vi "To XML - Invalid character in Message - XML does not contain invalid character.vi"() -> ()   [LabVIEW 2013, in "JUnit XML Tests.lvlib" / "Test Case.lvlib"]
uses:
  Test Case.lvlib
  JUnit XML/Test Case/Test Case.lvclass
  <vilib>/addons/_JKI Toolkits/Caraya/classes/Assert/Assert Equal Value_Variant.vi
  <vilib>/addons/_JKI Toolkits/Caraya/classes/Test/Test.lvclass
  <vilib>/addons/_JKI Toolkits/Caraya/classes/Assert/Assert.lvclass
panel:
  out "error out":errorcluster
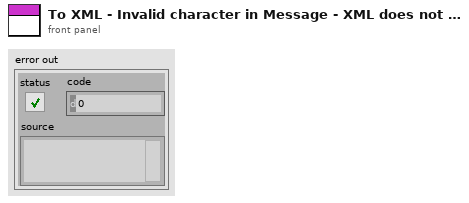
[diagram p1: front panel]
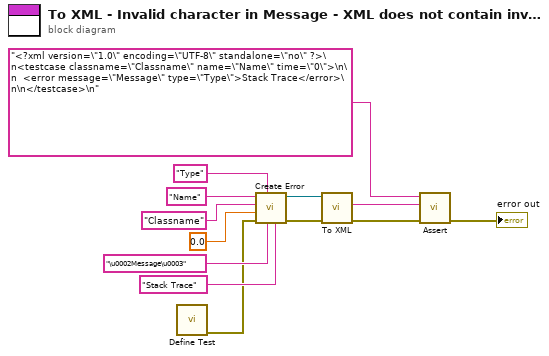
[diagram p0: block diagram]
diagram:
  n1 = call <vilib>:"Define Test.vi"() -> ("error out"=w1:errorcluster)  [unwired: 10 in, 1 out]
  n2 = call "Create Error.vi"("Stack Trace"="Stack Trace", "Message"="\u0002Message\u0003", "Type"="Type", "error in (no error)"=w1, "Time"=0.0, "Classname"="Classname", "Name"="Name") -> ("error out"=w12:errorcluster, "Test Case"=w13:refnum<class "Test Case.lvclass">)  [unwired: 3 in]
  n3 = call-dynamic "To XML.vi"("error in (no error)"=w12, "Serializable in"=w13) -> ("error out"=w2:errorcluster, "XML"=w3:string)  [unwired: 8 in]
  n4 = call-poly <vilib>:"Assert.vi"("error in (no error)"=w2, "Actual"=w3, "Expected"="<?xml version=\"1.0\" encoding=\"UTF-8\" standalone=\"no\" ?>\n<testcase classname=\"Classname\" name=\"Name\" time=\"0\">\n\n  <error message=\"Message\" type=\"Type\">Stack Trace</error>\n\n</testcase>\n") -> ("error out"=→"error out":errorcluster)  [unwired: 7 in, 1 out]
